vi "Write File Record.vi"(0 "MB session in":refnum<class "MB_Master.lvclass">, 5 "File Number":u16, 7 "Record Number":u16, 9 "values":u16[](array[numeric]), 11 "error in (no error)":errorcluster) -> (4 "MB session out":refnum<class "MB_Master.lvclass">, 15 "error out":errorcluster)   [LabVIEW 2016, in "斯坦道氨氮V2.lvlib"]
uses:
  <vilib>/Plasmionique/MB Master/MB_Master/MB_Master.lvclass
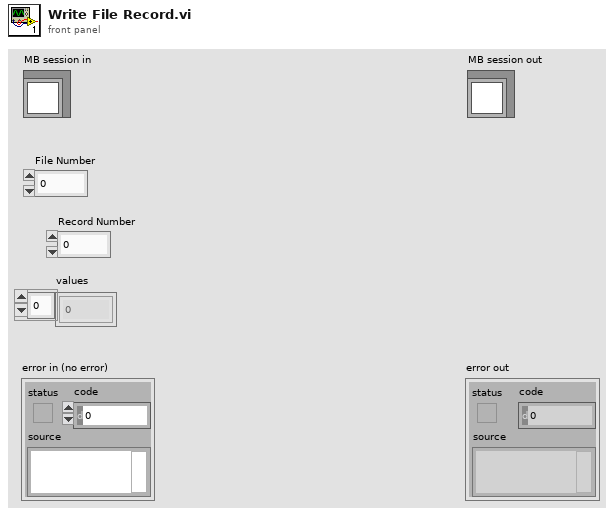
[diagram p1: front panel]
types:
  T1 = typedef "MB Master.lvlib/MB_PDU_Cluster.ctl" = cluster{"Function Code":u8, "Data":u8[], "RTU_DataBytes":i32}
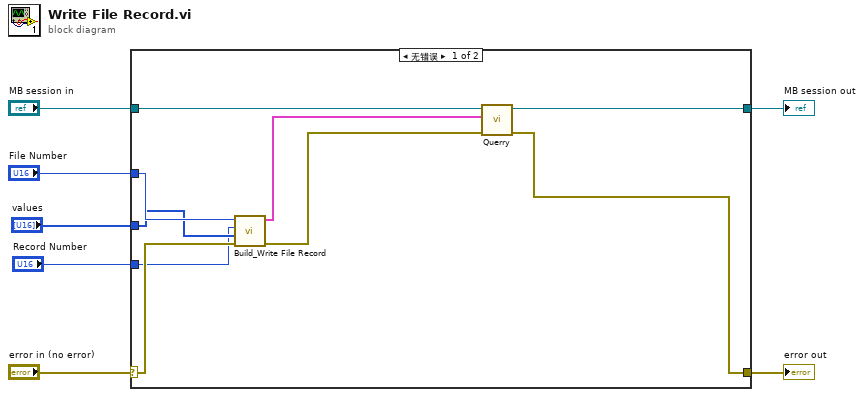
[diagram p0: block diagram]
diagram:
  n1 = case shown="无错误" "error in (no error)" {
    selector: "error in (no error)" -> [w11 w18]
    tunnel: [w15 w18] -> w6
    tunnel: [w16 w17] -> w4
    tunnel: "MB session in" -> [w14 w17]
    tunnel: "File Number" -> [w13 _]
    tunnel: "values" -> [w12 _]
    tunnel: "Record Number" -> [w8 _]
    frame No Error {
      n2 = call "Build_Write File Record.vi"("File Number"=w13, "Record Number"=w8, "values"=w12, "error in (no error)"=w11) -> ("MB_PDU"=w10:T1, "error out"=w9:errorcluster)  [unwired: 5 in]
      n3 = call-dynamic "Querry.vi"("error in (no error)"=w9, "PDU_req"=w10, "MB_Master in"=w14) -> ("error out"=w15:errorcluster, "MB_Master out"=w16:refnum<class "MB_Master.lvclass">)  [unwired: 6 in, 1 out]
    }
    frame Error {
    }
  }
  "error out" <- w6
  "MB session out" <- w4
